vi "SimpleSumVI.vi"(9 "Y":dbl, 11 "X":dbl) -> (3 "Result":dbl)   [LabVIEW 2023, in "SimpleClassInVi.lvclass"]
uses:
  SimpleClassInVi.lvclass
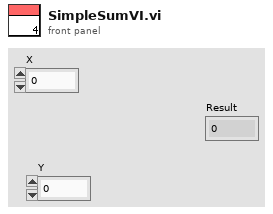
[diagram p1: front panel]
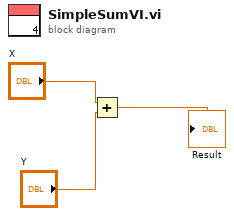
[diagram p0: block diagram]
diagram:
  n1 = Add(x="X", y="Y") -> (x+y=→"Result":dbl)
